vi "Get Window Rectangle.vi"(8 "error in":errorcluster {"code" format="%d\n%x"}, 10 "Visible Only? (T)":bool=TRUE, 11 "window refnum (NaWR)":T1) -> (0 "error out":errorcluster {"code" format="%d\n%x"}, 2 "window rect":T2, 3 "window refnum out":T1)   [LabVIEW 2020, in "MacroAssert.lvlib" / "Win Util.lvlib"]
doc: "This VI will find the coordinates of the upper left and lower right corners of the window identified by the 'window refnum' parameter. Coordinate values are in pixels, relative to the upper left corner of the screen. The 'window refnum' can be obtained by using 'Get Window RefNum.vi'."
uses:
  Win Util.lvlib
  Window Refnum.ctl
  user32.dll
  dwmapi.dll
  kernel32.dll
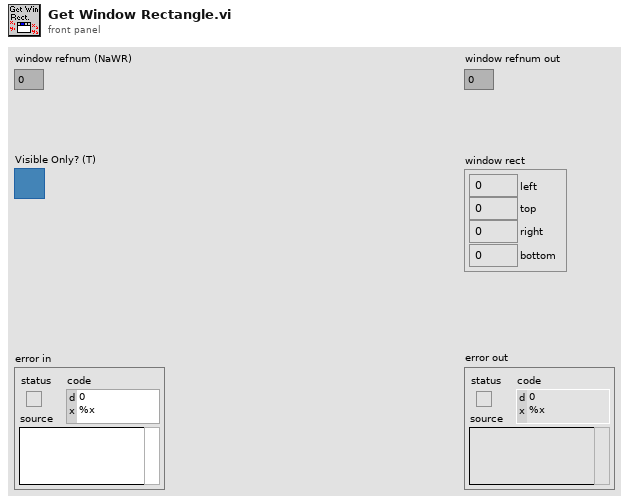
[diagram p1: front panel]
types:
  T1 = typedef "MacroAssert.lvlib/Win Util.lvlib/Window Refnum.ctl" = u64
  T2 = cluster{"left":i16, "top":i16, "right":i16, "bottom":i16}
  T3 = cluster{"RECT[0]":i32, "RECT[1]":i32, "RECT[2]":i32, "RECT[3]":i32}
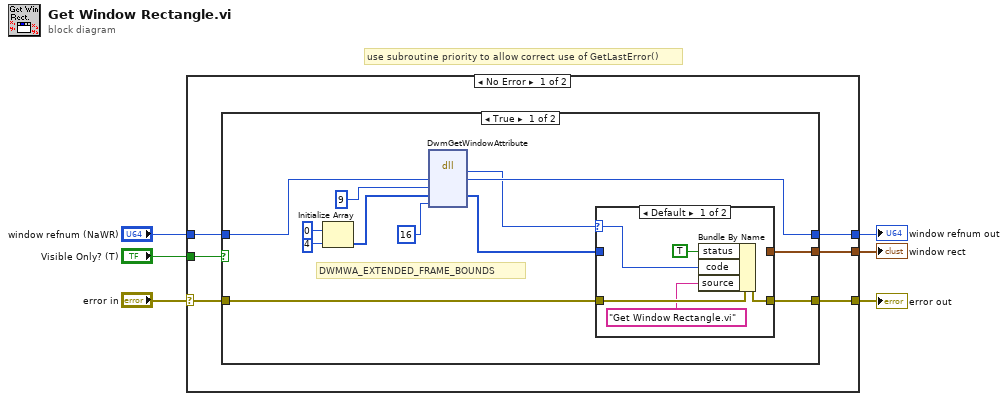
[diagram p0: block diagram]
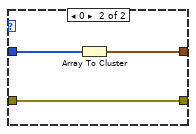
[diagram p2: hidden frame]
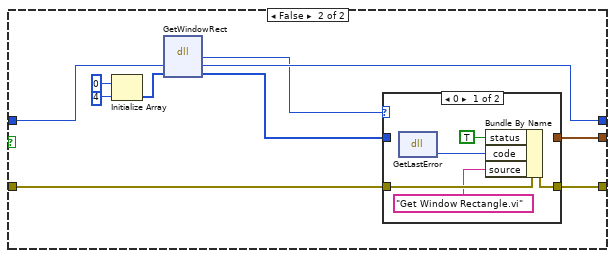
[diagram p3: hidden frame]
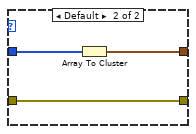
[diagram p4: hidden frame]
diagram:
  # "use subroutine priority to allow correct use of GetLastError()"
  n1 = case shown="No Error" "error in" {
    selector: "error in" -> [w9 w52]
    tunnel: [w10 w51] -> w4
    tunnel: [w8 w52] -> w6
    tunnel: "window refnum (NaWR)" -> [w11 w51]
    tunnel: [w12 _] -> w3
    tunnel: "Visible Only? (T)" -> [w7 _]
    frame No Error {
      n2 = case shown="True" w7 {
        tunnel: [w23 w41] -> w12
        tunnel: w11 -> [w22 w40]
        tunnel: [w21 w39] -> w10
        tunnel: w9 -> [w19 w37]
        tunnel: [w18 w36] -> w8
        frame True {
          # "DWMWA_EXTENDED_FRAME_BOUNDS"
          n3 = Initialize Array(0, 4) -> (w15:i32[])
          n4 = dll-call lib="dwmapi.dll" fn="DwmGetWindowAttribute"("hWnd"=w22, "dwAttribute"=9, "RECT"=w15, "cbAttribute"=16 ("dwAttribute")) -> ("Return Value"=w20:i32, "hWnd"=w21:u64, "RECT"=w24:i32[])  [unwired: 4 in, 3 out]
          n5 = case shown="Default" w20 {
            selector: w20 -> [w25 _]
            tunnel: w24 -> [_ w32]
            tunnel: [_ w31] -> w23
            tunnel: w19 -> [w29 w30]
            tunnel: [w28 w30] -> w18
            frame Default {
              n6 = Bundle By Name(cluster=w29, "status"=TRUE ("show call chain? (False)"), "code"=w25, "source"="Get Window Rectangle.vi") -> (w28:errorcluster)
            }
            frame 0 {
              n7 = Array To Cluster(array=w32) -> (cluster=w31:T3)
            }
          }
        }
        frame False {
          n8 = Initialize Array(0, 4) -> (w33:i32[])
          n9 = dll-call lib="USER32.DLL" fn="GetWindowRect"("hWnd"=w40, "RECT"=w33) -> ("Return Value"=w38:i32, "hWnd"=w39:u64, "RECT"=w42:i32[])  [unwired: 3 in, 2 out]
          n10 = case shown="0" w38 {
            tunnel: w42 -> [_ w50]
            tunnel: [_ w49] -> w41
            tunnel: w37 -> [w47 w48]
            tunnel: [w46 w48] -> w36
            frame 0 {
              n11 = dll-call lib="kernel32.dll" fn="GetLastError"() -> ("return type"=w44:i32)  [unwired: 3 in, 2 out]
              n12 = Bundle By Name(cluster=w47, "status"=TRUE ("show call chain? (False)"), "code"=w44, "source"="Get Window Rectangle.vi") -> (w46:errorcluster)
            }
            frame Default {
              n13 = Array To Cluster(array=w50) -> (cluster=w49:T3)
            }
          }
        }
      }
    }
    frame Error {
    }
  }
  "error out" <- w6
  "window refnum out" <- w4
  "window rect" <- w3
